vi "Write Listbox Header.vi"(8 "error in":errorcluster, 10 "Value":string, 11 "Listbox Ref in":refnum<vi>) -> (0 "error out":errorcluster, 3 "Listbox Ref out":refnum<vi>)   [LabVIEW 2020, in "G-Unicode.lvlib"]
uses:
  Unicode/Controls/String Encoding.ctl
  G-Unicode.lvlib
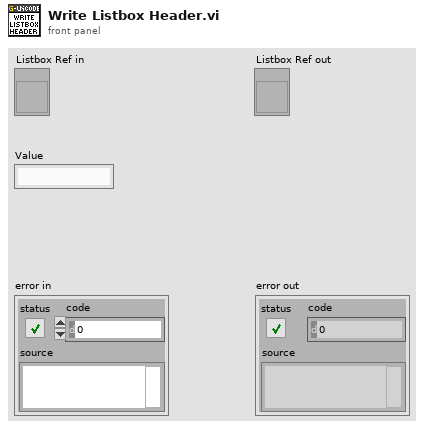
[diagram p1: front panel]
types:
  T1 = typedef "G-Unicode.lvlib/String Encoding.ctl" = enum16{"ANSI", "UTF-8", "UTF-16LE", "UTF-16BE", "Unknown"}
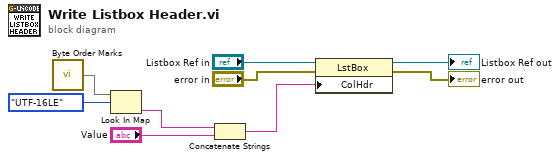
[diagram p0: block diagram]
diagram:
  n1 = call "Byte Order Marks.vi"() -> ("BOMs"=w5:map{T1, string})
  n2 = Look In Map(map=w5, key=String_Encoding."UTF-16LE") -> (value=w3:string)  [unwired: 1 in, 1 out]
  n3 = Concatenate Strings(w3, "Value") -> (w1:string)
  n4 = property class="LstBox"(reference="Listbox Ref in", error in="error in", "ColHdr"=w1) -> (reference out=→"Listbox Ref out":refnum<vi>, error out=→"error out":errorcluster)
